vi "Version3.2.vi"() -> ()   [LabVIEW 2012]
uses:
  <vilib>/Instr/_visa.llb/VISA Configure Serial Port (Instr).vi
  Function_Set/Debug/Function_Set.dll
panel:
  in  "选项卡控件":enum32{"Note", "AVT CCD", "Vacuum REC", "..."}(tab)
  in  "Double:":dbl
  in  "String:":string
  in  "Other:":string
  in  "Save This Shot":bool
  out "Shots:":i32
  in  "Save This Notes":bool
  in  "Other Notes:":string
  out "Shot's situation:":string
  out "Shots: 2":i32
  out "Notes:":string
  in  "查询":bool
  in  "Options":u16(ring) caption="Choose File:"
  in  "Initial Folder Path:":path
  in  "Your Own:":u16(ring) items=["2, 0, 3, 2"]
  in  "FrameStartTriggerMode":T1(ring)
  in  "AcquisitionMode":T2(ring)
  in  "ExposureMode":T3(ring)
  in  "AVT SDK Demon":bool
  out "CCD ID":string
  out "ExposureMode":string
  out "ExposureValue":u32
  out "AcquisitionMode":string
  out "FrameStartTriggerMode":string
  in  "ExposureValue":u32
  in  "CameraStart":bool
  in  "CameraStop":bool
  in  "CameraSet":bool
  in  "CameraGet":bool
  in  "CameraSetAll":bool
  in  "path to JPEG file":path caption="Path of the Pic"
  out "new picture":picture caption="Pic"
  in  "OPEN":bool
  in  "端口选择":refnum<visa-resource-name>="COM1"
  in  "baud rate":u32=9600
  in  "data bits":u16=8
  in  "stop bits":u16(ring)=10 items=["1.0"=10, "1.5"=15, "2.0"=20]
  in  "flow control":u16(ring) items=["None"=0, "XON/XOFF"=1, "RTS/CTS"=2, "DTR/DSR"=4]
  in  "timeout":u32=10
  in  "RS485地址":string="12"
  in  "读取间隔(s)":dbl=1.0 caption="Delay Time (s)"
  in  "数据文件夹":string="data"
  in  "记录说明":string="test"
  out "数据路径":path
  in  "parity (0:none)":enum16{"None", "Odd", "Even", "Mark", "Space"}(ring)
  in  "记录所有读取数据?":bool
  out "已记录数据点":u32 caption="recorded number"
  in  "stop":bool
  out "电离规图表":dbl(graph)
  out "电阻规图表":dbl(graph)
  out "已读取数据点":i32
  out "预定耗时":dbl
  out "实际耗时":dbl
  in  "临界压强(Pa)":dbl=8.0
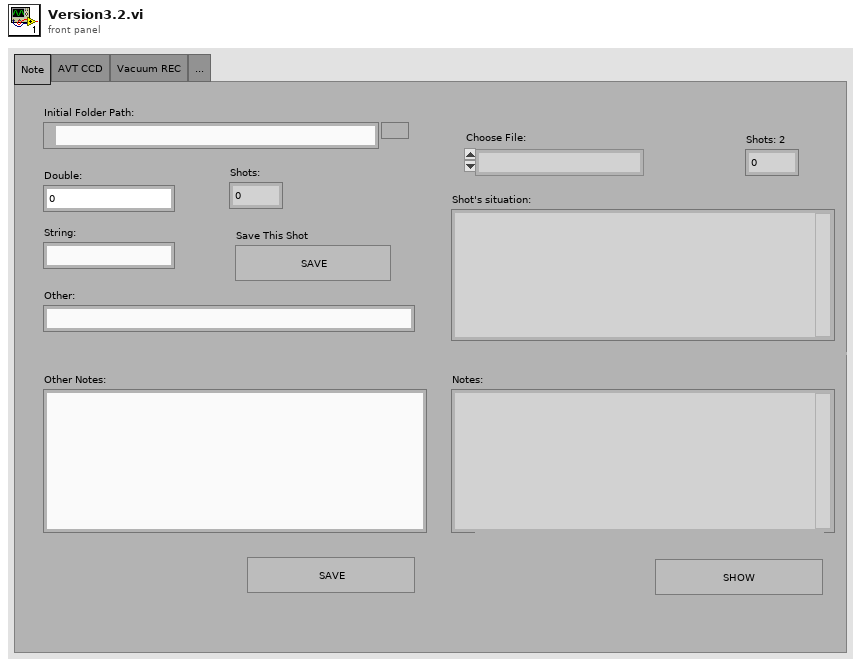
[diagram p1: front panel]
types:
  T1 = enum16{"默认", "Freerun", "SyncIn1", "SyncIn2", "FixedRate", "Software"}
  T2 = enum16{"默认", "Continuous", "SingleFrame", "MultiFrame", "Recorder"}
  T3 = enum16{"默认", "Manual", "Auto", "AutoOnce", "External"}
  T4 = enum32{"Record", "Instrument 1", "Instrument 2", "..."}
  T5 = enum16{"open", "replace", "create", "open or create", "replace or create", "replace or create with confirmation"}
  T6 = typedef "imagedata.ctl" = cluster{"image type":i32, "image depth":i32, "image":u8[], "mask":u8[], "colors":u32[], "Rectangle":cluster{"left":i16, "top":i16, "right":i16, "bottom":i16}}
  T7 = cluster{"Resister":dbl, "Ionization":dbl, "time":string, "Ionization":dbl, "Ionization":dbl, u32, i32}
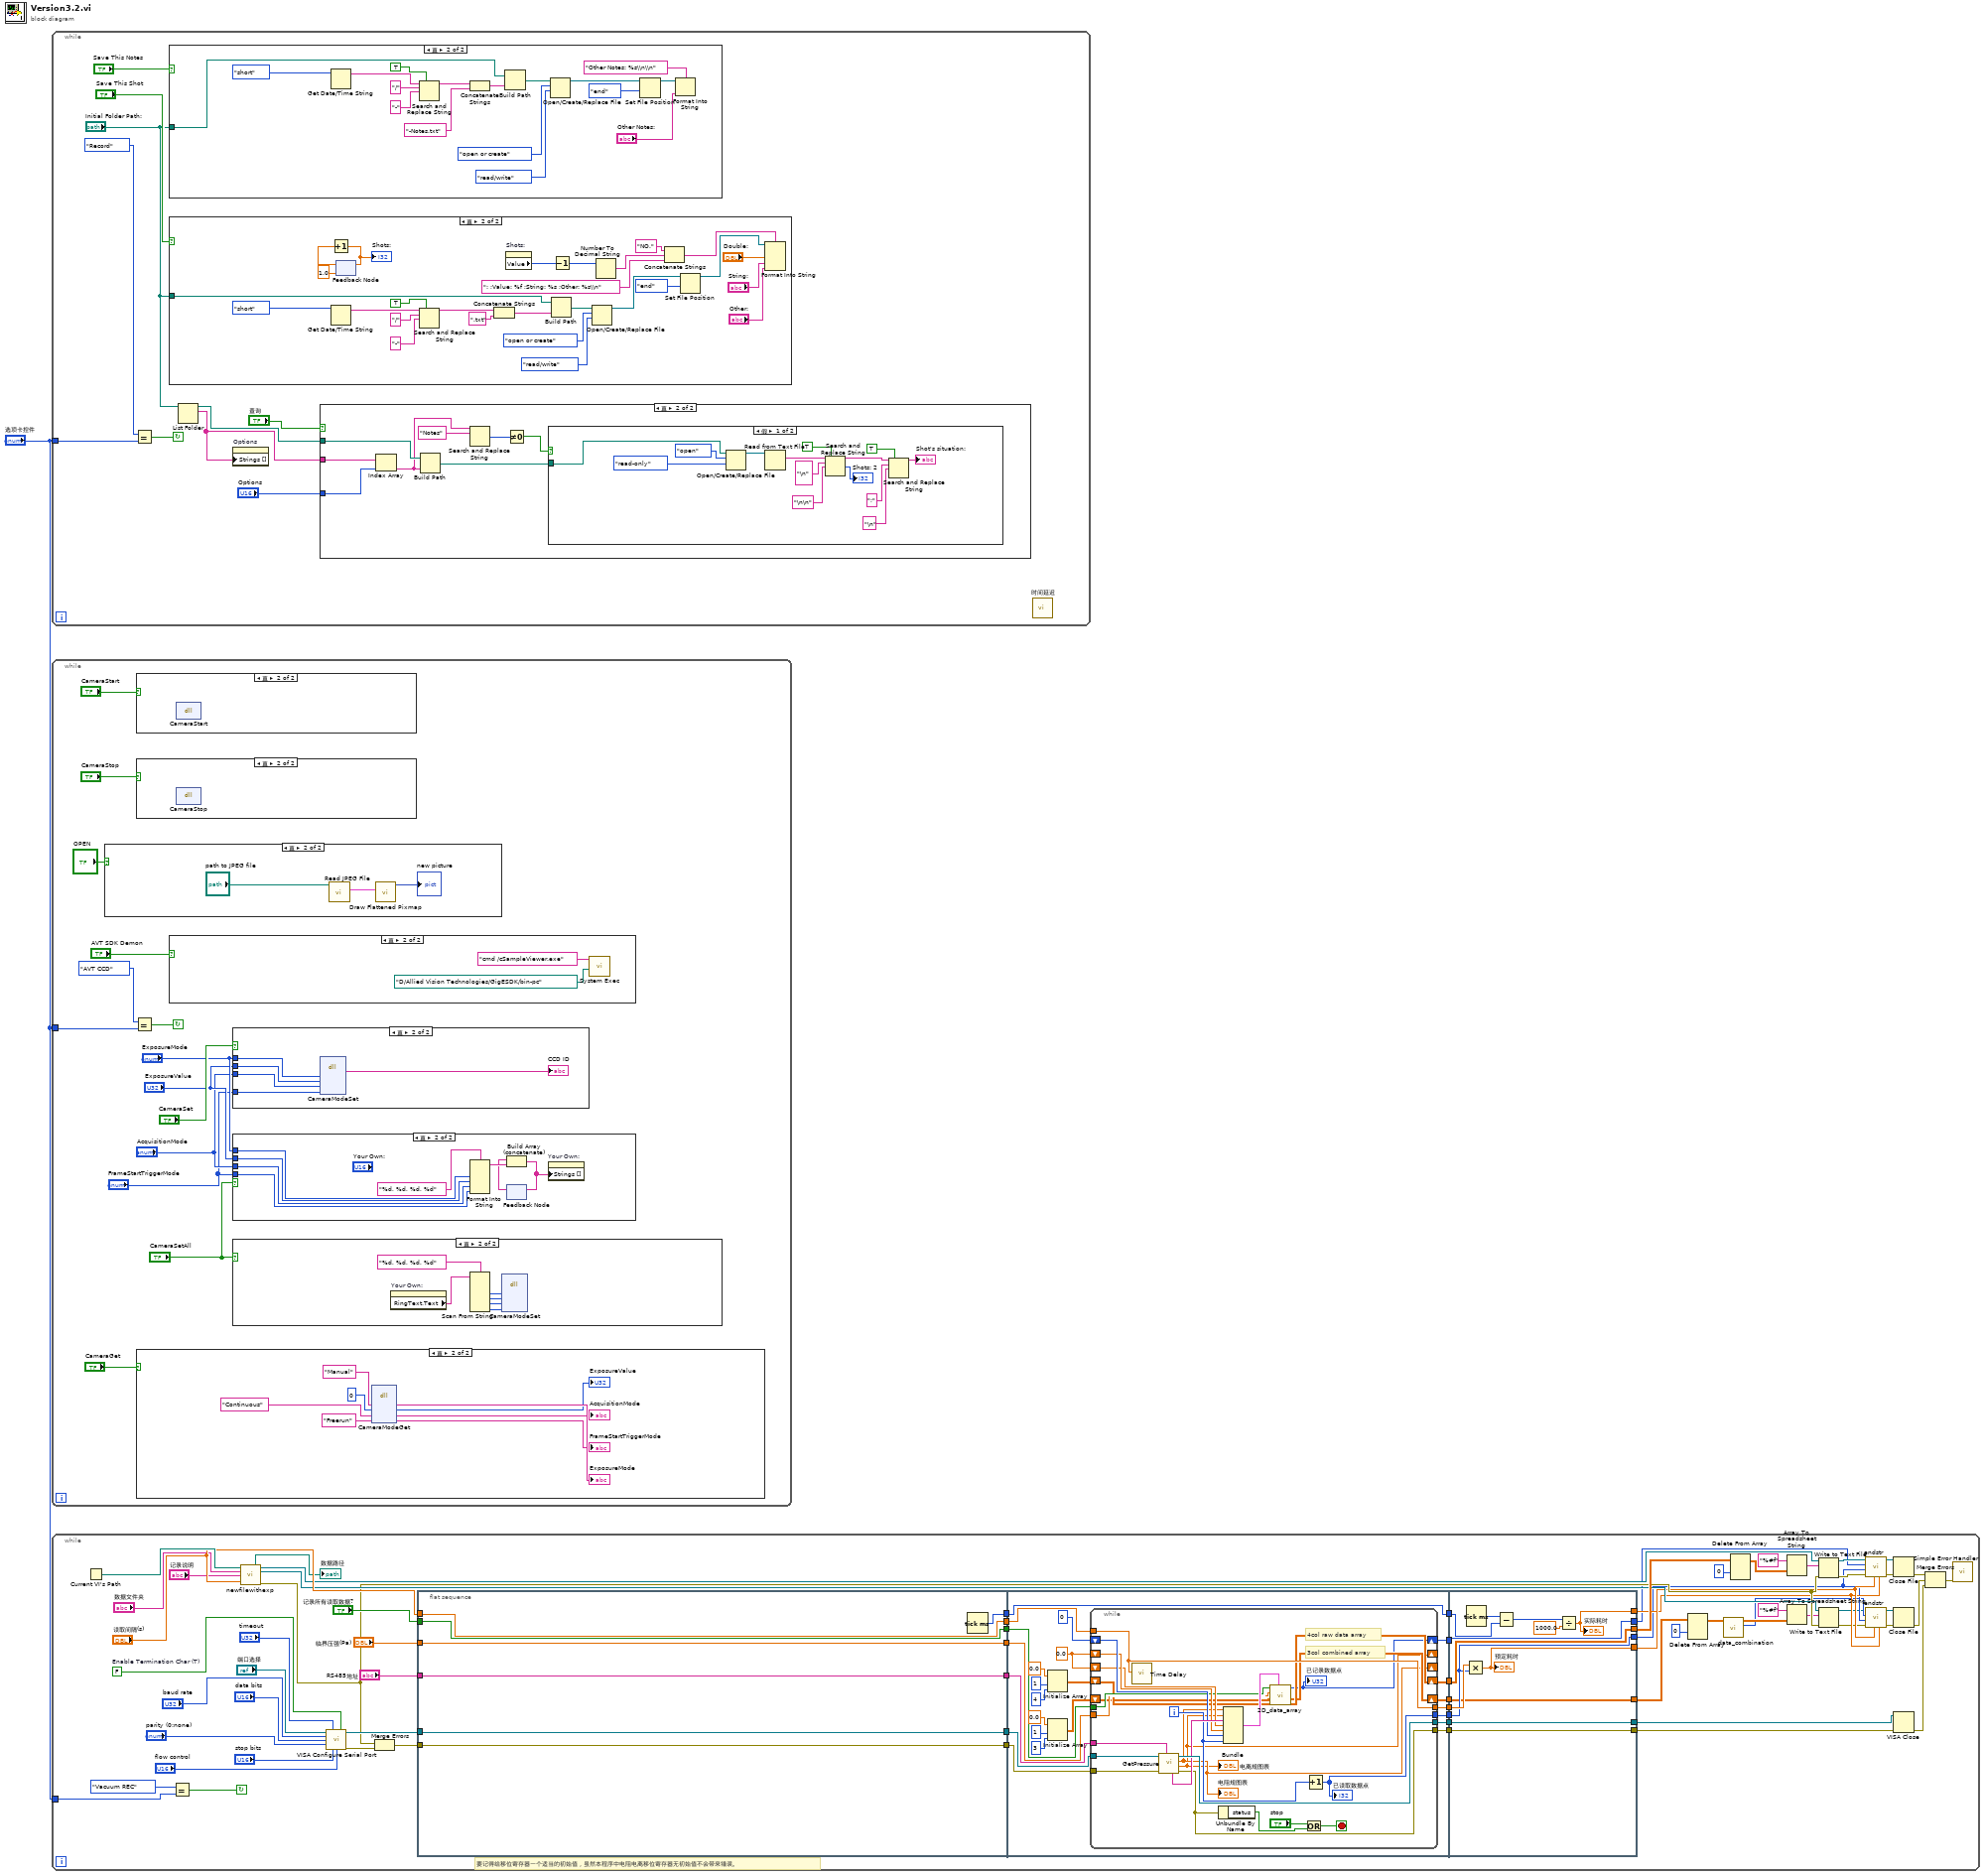
[diagram p0: block diagram]
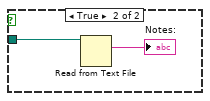
[diagram p11: hidden frame]
diagram:
  n1 = while {
    tunnel: "选项卡控件" -> [w4]
    stop <- w5 continue-if-true
    n2 = Equal?(x=T4."Record", y=w4) -> (x = y?=w5:bool)
    n3 = case shown="真" "Save This Notes" {
      tunnel: "Initial Folder Path:" -> [_ w36]
      frame False {
      }
      frame True {
        n4 = Get Date/Time String(date format (0)=enum16{"short", "long", "abbreviated"}."short" ("日期格式(0)")) -> (date string=w48:string)  [unwired: 2 in, 1 out]
        n5 = Search and Replace String(replace all?=TRUE ("替换全部？(F)"), input string=w48, search string="/" ("搜索字符串"), replace string="-" ("替换字符串(\"\")")) -> (result string=w39:string)  [unwired: 4 in, 3 out]
        n6 = Concatenate Strings(w39, "-Notes.txt" ("字符串")) -> (w37:string)
        n7 = Build Path(base path=w36, name or relative path=w37) -> (appended path=w49:path)
        n8 = Open/Create/Replace File(file path (use dialog)=w49, operation (0:open)=T5."open or create" ("操作(0:open)"), access (0:read/write)=enum16{"read/write", "read-only", "write-only"}."read/write" ("权限(0:read/write)")) -> (refnum out=w42:refnum<file>)  [unwired: 3 in, 2 out]
        n9 = Set File Position(refnum=w42, from (0:start)=enum16{"start", "end", "current"}."end" ("自（0:起始）")) -> (refnum out=w41:refnum<file>)  [unwired: 2 in, 1 out]
        n10 = Format Into String(format string="Other Notes: %s\\n\\n" ("格式字符串"), initial string=w41, "Other Notes:") -> ()  [unwired: 1 in, 2 out]
      }
    }
    n11 = case shown="真" "Save This Shot" {
      tunnel: "Initial Folder Path:" -> [_ w59]
      frame False {
      }
      frame True {
        n12 = Get Date/Time String(date format (0)=enum16{"short", "long", "abbreviated"}."short" ("日期格式(0)")) -> (date string=w73:string)  [unwired: 2 in, 1 out]
        n13 = feedback #1(1.0 ("x")) -> (w62:dbl)
        n14 = Increment(x=w62) -> (x+1=w60:dbl)
        "Shots:" <- w60
        n15 = feedback-in #1(w60) -> ()
        n16 = Search and Replace String(replace all?=TRUE ("替换全部？(F)"), input string=w73, search string="/" ("搜索字符串"), replace string="-" ("替换字符串(\"\")")) -> (result string=w70:string)  [unwired: 4 in, 3 out]
        n17 = Concatenate Strings(w70, ".txt" ("字符串")) -> (w75:string)
        n18 = property on="Shots:" class="DigNum (严格)"() -> ("Value"=w54:i32)  [unwired: 2 in, 2 out]
        n19 = Build Path(base path=w59, name or relative path=w75) -> (appended path=w76:path)
        n20 = Decrement(x=w54) -> (x-1=w53:i32)
        n21 = Open/Create/Replace File(file path (use dialog)=w76, operation (0:open)=T5."open or create" ("操作(0:open)"), access (0:read/write)=enum16{"read/write", "read-only", "write-only"}."read/write" ("权限(0:read/write)")) -> (refnum out=w64:refnum<file>)  [unwired: 3 in, 2 out]
        n22 = Number To Decimal String(number=w53) -> (decimal integer string=w58:string)  [unwired: 1 in]
        n23 = Concatenate Strings("NO." ("字符串"), w58, ": ;Value: %f ;String: %s ;Other: %s\\n" ("格式字符串")) -> (w55:string)
        n24 = Set File Position(refnum=w64, from (0:start)=enum16{"start", "end", "current"}."end" ("自（0:起始）")) -> (refnum out=w63:refnum<file>)  [unwired: 2 in, 1 out]
        n25 = Format Into String(format string=w55, initial string=w63, "Double:", "String:", "Other:") -> ()  [unwired: 1 in, 2 out]
      }
    }
    n26 = List Folder(path="Initial Folder Path:") -> (path out=w8:path, filenames=w6:string[])  [unwired: 3 in, 2 out]
    n27 = property on="Options" class="Ring (严格)"("Strings []"=w6) -> ()  [unwired: 2 in, 2 out]
    n28 = case shown="真" "查询" {
      tunnel: w6 -> [_ w19]
      tunnel: "Options" -> [_ w18]
      tunnel: w8 -> [_ w17]
      frame False {
      }
      frame True {
        n29 = Index Array(array=w19, index=w18) -> (element=w16:string)
        n30 = Build Path(base path=w17, name or relative path=w16) -> (appended path=w12:path)
        n31 = Search and Replace String(input string=w16, search string="Notes" ("搜索字符串")) -> (number of replacements=w14:i32)  [unwired: 6 in, 3 out]
        n32 = Not Equal To 0?(x=w14) -> (x != 0?=w13:bool)
        n33 = case shown="假" w13 {
          tunnel: w12 -> [w33 w35]
          frame False {
            n34 = Open/Create/Replace File(file path (use dialog)=w33, operation (0:open)=T5."open" ("操作(0:open)"), access (0:read/write)=enum16{"read/write", "read-only", "write-only"}."read-only" ("权限(0:read/write)")) -> (refnum out=w30:refnum<file>)  [unwired: 3 in, 2 out]
            n35 = Read from Text File(file (use dialog)=w30) -> (text=w26:string)  [unwired: 3 in, 3 out]
            n36 = Search and Replace String(replace all?=TRUE ("替换全部？(F)"), input string=w26, search string="\n" ("搜索字符串"), replace string="\n\n" ("替换字符串(\"\")")) -> (result string=w23:string, number of replacements=→"Shots: 2":i32)  [unwired: 4 in, 2 out]
            n37 = Search and Replace String(replace all?=TRUE ("替换全部？(F)"), input string=w23, search string=";" ("搜索字符串"), replace string="\n" ("替换字符串(\"\")")) -> (result string=→"Shot's situation:":string)  [unwired: 4 in, 3 out]
          }
          frame True {
            n38 = Read from Text File(file (use dialog)=w35) -> (text=→"Notes:":string)  [unwired: 3 in, 3 out]
          }
        }
      }
    }
    n39 = call "时间延迟"() -> ()  [unwired: 11 in, 1 out]
  }
  n40 = while {
    tunnel: "选项卡控件" -> [w83]
    stop <- w84 continue-if-true
    n41 = case shown="真" "OPEN" {
      frame False {
      }
      frame True {
        n42 = call <vilib>:"Read JPEG File.vi"("path to JPEG file"="path to JPEG file") -> ("image data"=w94:T6)  [unwired: 8 in, 2 out]
        n43 = call <vilib>:"Draw Flattened Pixmap.vi"("image data"=w94) -> ("new picture"=→"new picture":picture)  [unwired: 8 in]
      }
    }
    n44 = Equal?(x=enum32{"Note", "AVT CCD", "Vacuum REC", "..."}."AVT CCD", y=w83) -> (x = y?=w84:bool)
    n45 = case shown="真" "CameraStart" {
      frame False {
      }
      frame True {
        n46 = dll-call lib="F:/Kun's Test/Function_Set/Debug/Function_Set.dll" fn="CameraStart"() -> ()  [unwired: 4 in, 2 out]
      }
    }
    n47 = case shown="真" "CameraStop" {
      frame False {
      }
      frame True {
        n48 = dll-call lib="F:/Kun's Test/Function_Set/Debug/Function_Set.dll" fn="CameraStop"() -> ()  [unwired: 4 in, 2 out]
      }
    }
    n49 = case shown="真" "CameraGet" {
      frame False {
      }
      frame True {
        n50 = dll-call lib="F:/Kun's Test/Function_Set/Debug/Function_Set.dll" fn="CameraModeGet"("ExposureMode"="Manual", "ExposureValue"=u32 0, "AcquisitionMode"="Continuous", "FrameStartTriggerMode"="Freerun") -> ("ExposureMode"=→"ExposureMode":string, "ExposureValue"=→"ExposureValue":u32, "AcquisitionMode"=→"AcquisitionMode":string, "FrameStartTriggerMode"=→"FrameStartTriggerMode":string)  [unwired: 4 in, 2 out]
      }
    }
    n51 = case shown="真" "AVT SDK Demon" {
      frame False {
      }
      frame True {
        n52 = call <vilib>:"System Exec.vi"("working directory"=path "D:/Allied Vision Technologies/GigESDK/bin-pc", "command line"="cmd /cSampleViewer.exe") -> ()  [unwired: 6 in, 4 out]
      }
    }
    n53 = case shown="真" "CameraSet" {
      tunnel: "ExposureValue" -> [_ w122]
      tunnel: "ExposureMode" -> [_ w121]
      tunnel: "AcquisitionMode" -> [_ w120]
      tunnel: "FrameStartTriggerMode" -> [_ w119]
      frame False {
      }
      frame True {
        n54 = dll-call lib="F:/Kun's Test/Function_Set/Debug/Function_Set.dll" fn="CameraModeSet"("EM"=w121, "EV"=w122, "AM"=w120, "FSTM"=w119) -> ("返回类型"=→"CCD ID":string)  [unwired: 7 in, 2 out]
      }
    }
    n55 = case shown="真" "CameraSetAll" {
      tunnel: "ExposureMode" -> [_ w106]
      tunnel: "ExposureValue" -> [_ w105]
      tunnel: "AcquisitionMode" -> [_ w104]
      tunnel: "FrameStartTriggerMode" -> [_ w103]
      frame False {
      }
      frame True {
        n56 = Format Into String(format string="%d, %d, %d, %d" ("格式字符串"), w106, w105, w104, w103) -> (resulting string=w109:string)  [unwired: 2 in, 1 out]
        n57 = feedback #2() -> (w108:string[])  [unwired: 1 in]
        n58 = Build Array (concatenate)(w108, w109) -> (w107:string[])
        n59 = feedback-in #2(w107) -> ()
        n60 = property on="Your Own:" class="Ring (严格)"("Strings []"=w107) -> ()  [unwired: 2 in, 2 out]
      }
    }
    n61 = case shown="真" "CameraSetAll" {
      frame False {
      }
      frame True {
        n62 = property on="Your Own:" class="Ring (严格)"() -> ("RingText.Text"=w97:string)  [unwired: 2 in, 2 out]
        n63 = Scan From String(format string="%d, %d, %d, %d" ("格式字符串"), input string=w97) -> (output 1=w99:i32, output 2=w100:i32, output 3=w101:i32, output 4=w102:i32)  [unwired: 6 in, 3 out]
        n64 = dll-call lib="F:/Kun's Test/Function_Set/Debug/Function_Set.dll" fn="CameraModeSet"("EM"=w99, "EV"=w100, "AM"=w101, "FSTM"=w102) -> ()  [unwired: 8 in, 2 out]
      }
    }
  }
  n65 = while {
    tunnel: "选项卡控件" -> [w127]
    stop <- w128 continue-if-true
    w178 = FALSE  # Enable Termination Char (T)
    # "要记得给移位寄存器一个适当的初始值，虽然本程序中电阻电离移位寄存器无初始值不会带来错误。"
    n66 = Current VI's Path() -> (path=w170:path)
    n67 = Equal?(x=enum32{"Note", "AVT CCD", "Vacuum REC", "..."}."Vacuum REC", y=w127) -> (x = y?=w128:bool)
    n68 = call "newfilewithexp.vi"("路径"=w170, "数据文件夹"="数据文件夹", "记录说明"="记录说明", "读取间隔(s)"="读取间隔(s)") -> ("数据路径"=→"数据路径":path, "refnum out for 4column"=w149:refnum<file>, "refnum out for 3column"=w147:refnum<file>, "error out"=w146:errorcluster)  [unwired: 1 in, 7 out]
    n69 = call-poly "VISA Configure Serial Port"("VISA resource name"="端口选择", "timeout (10sec)"="timeout", "Enable Termination\nChar (T)"=w178, "baud rate (9600)"="baud rate", "data bits (8)"="data bits", "parity (0:none)"="parity (0:none)", "stop bits (10: 1 bit)"="stop bits", "flow control (0:none)"="flow control") -> ("VISA resource name out"=w175:refnum<visa-resource-name>, "error out"=w150:errorcluster)  [unwired: 1 in, 5 out]
    n70 = Merge Errors(w146, w150) -> (w158:errorcluster)
    n71 = flat-sequence {
      tunnel: "RS485地址" -> [w198]
      tunnel: "读取间隔(s)" -> [w199]
      tunnel: "记录所有读取数据?" -> [w200]
      tunnel: w158 -> [w201]
      tunnel: w175 -> [w202]
      tunnel: [w202] -> w195
      tunnel: [w201] -> w194
      tunnel: [w200] -> w193
      tunnel: [w199] -> w192
      tunnel: [w198] -> w191
      tunnel: [w197] -> w190
      tunnel: "临界压强(Pa)" -> [w196]
      tunnel: [w196] -> w189
      tunnel: [w224] -> w188
      tunnel: [w203] -> w187
      tunnel: w195 -> [w226]
      tunnel: w194 -> [w225]
      tunnel: w193 -> [w222]
      tunnel: w192 -> [w221]
      tunnel: w191 -> [w220]
      tunnel: [w219] -> w186
      tunnel: w190 -> [w219]
      tunnel: [w218] -> w185
      tunnel: [w217] -> w184
      tunnel: w189 -> [w216]
      tunnel: [w215] -> w183
      tunnel: [w209] -> w182
      tunnel: [w204] -> w181
      tunnel: [w263] -> w173
      tunnel: [w264] -> w174
      tunnel: w188 -> [w264]
      tunnel: w187 -> [w263]
      tunnel: w186 -> [w261]
      tunnel: w185 -> [w255]
      tunnel: w184 -> [w258]
      tunnel: w183 -> [w256]
      tunnel: w182 -> [w257]
      tunnel: [w257] -> w163
      tunnel: [w256] -> w142
      tunnel: [w255] -> w141
      tunnel: [w254] -> w144
      tunnel: [w253] -> w143
      tunnel: w181 -> [w252]
      tunnel: [w252] -> w157
      frame #0 {
        n72 = Tick Count (ms)() -> (millisecond timer value=w197:u32)
      }
      frame #1 {
        w214 = 0.0 ("Ionization")
        n73 = Initialize Array(0.0 ("element"), 1 ("dimension size"), 4 ("dimension size")) -> (w212:dbl[][])
        n74 = Initialize Array(0.0 ("element"), 1 ("dimension size"), 3 ("dimension size")) -> (w205:dbl[][])
        n75 = while {
          tunnel: w226 -> [w251]
          tunnel: w225 -> [w250]
          tunnel: w220 -> [w247]
          tunnel: [w233] -> w224
          tunnel: [w248] -> w203
          shift-right: [w234] -> w215
          shift-left: u32 0 -> [w244]
          shift-right: [w228] -> _
          shift-left: w214 -> [w243]
          tunnel: w221 -> [w249]
          tunnel: w222 -> [w240]
          tunnel: [w227] -> w218
          tunnel: [w249] -> w217
          shift-right: [w229] -> _
          shift-left: w214 -> [w242]
          tunnel: w216 -> [w239]
          shift-right: [w237] -> w209
          shift-left: w212 -> [w238]
          shift-right: [w235] -> w204
          shift-left: w205 -> [w236]
          i -> [w245]
          stop <- w230 stop-if-true
          # "4col raw data array"
          # "3col combined array"
          n76 = call "Time Delay"("Delay Time (s)"=w249) -> ()  [unwired: 1 in, 10 out]
          n77 = call "GetPressure.vi"("Address of RS485"=w247, "error in (no error)"=w250, "VISA resource name"=w251) -> ("error out"=w233:errorcluster, "Ionization"=w228:dbl, "Resister"=w229:dbl, "VISA resource name out"=w248:refnum<visa-resource-name>, "time"=w246:string)  [unwired: 1 in, 3 out]
          "电阻规图表" <- w229
          "电离规图表" <- w228
          n78 = Unbundle By Name(w233) -> ("status"=w231:bool)
          n79 = Bundle("Resister"=w229, "Ionization"=w228, "time"=w246, "Ionization"=w242, "Ionization"=w243, w244, w245) -> (w241:T7)  [unwired: 1 out]
          n80 = call "2D_data_array.vi"("input cluster"=w241, "input 4column array"=w238, "input combined 3column array"=w236, "critical pressure"=w239, "record all data points?"=w240) -> ("output 4column array"=w237:dbl[][], "output combined 3column array"=w235:dbl[][], "recorded number out"=w234:u32)  [unwired: 4 out]
          "已记录数据点" <- w234
          n81 = Or(x="stop", y=w231) -> (x .or. y?=w230:bool)
          n82 = Increment(x=w245) -> (x+1=w227:i32)
          "已读取数据点" <- w227
        }
      }
      frame #2 {
        n83 = Multiply(x=w258, y=w255) -> (x*y=w254:dbl)
        "预定耗时" <- w254
        n84 = Tick Count (ms)() -> (millisecond timer value=w262:u32)
        n85 = Subtract(x=w262, y=w261) -> (x-y=w260:u32)
        n86 = Divide(x=w260, y=1000.0) -> (x/y=w253:dbl)
        "实际耗时" <- w253
      }
    }
    n87 = Delete From Array(array=w157, index (row)=0) -> (array with subset deleted=w154:dbl[][])  [unwired: 2 in, 1 out]
    n88 = call "data_combination.vi"("input combined data array"=w154) -> ("recorded combined data number"=w140:i32, "output combined data array"=w151:dbl[][])  [unwired: 9 out]
    n89 = Delete From Array(array=w163, index (row)=0) -> (array with subset deleted=w164:dbl[][])  [unwired: 2 in, 1 out]
    n90 = Array To Spreadsheet String(array=w164, 3:"%#f" ("format string")) -> (spreadsheet string=w148:string)  [unwired: 1 out]
    n91 = Array To Spreadsheet String(array=w151, 3:"%#f" ("format string")) -> (spreadsheet string=w145:string)  [unwired: 1 out]
    n92 = Write to Text File(file (use dialog)=w149, text=w148, error in=w146) -> (refnum out=w160:refnum<file>, error out=w159:errorcluster)  [unwired: 2 out]
    n93 = Write to Text File(file (use dialog)=w147, text=w145, error in=w146) -> (refnum out=w139:refnum<file>, error out=w138:errorcluster)  [unwired: 2 out]
    n94 = call "endstr.vi"("实际耗时"=w143, "预定耗时"=w144, "error in"=w159, "已读取数据点"=w141, "已记录数据点"=w142, "refnum in"=w160) -> ("error out"=w162:errorcluster, "refnum out"=w161:refnum<file>)  [unwired: 4 out]
    n95 = call "endstr.vi"("实际耗时"=w143, "预定耗时"=w144, "error in"=w138, "已读取数据点"=w141, "已记录数据点"=w140, "refnum in"=w139) -> ("error out"=w152:errorcluster, "refnum out"=w153:refnum<file>)  [unwired: 4 out]
    n96 = Close File(refnum=w161, error in=w162) -> (error out=w134:errorcluster)  [unwired: 1 out]
    n97 = Close File(refnum=w153, error in=w152) -> (error out=w135:errorcluster)  [unwired: 1 out]
    n98 = VISA Close(VISA resource name=w173, error in (no error)=w174) -> (error out=w136:errorcluster)
    n99 = Merge Errors(w134, w135, w136) -> (w137:errorcluster)
    n100 = call <vilib>:"Simple Error Handler.vi"("error in (no error)"=w137) -> ()  [unwired: 1 in, 8 out]
  }
